vi "Run.vi"(8 "error in (no error)":errorcluster, 9 "s on last turn":dbl, 10 "Maze (0: Empty, -1: Enemy. >0: Teammate":i32[][](array[numeric]), 11 "Expand in":refnum<class "Hungry Wolf.lvclass">) -> (0 "error out":errorcluster, 1 "Direction":T1, 2 "Action":T2, 3 "Expand out":refnum<class "Hungry Wolf.lvclass">, 4 "Replicated":refnum<class "Square.lvclass">)   [LabVIEW 2015, in "Hungry Wolf.lvclass"]
uses:
  Hungry Wolf.lvclass
  Type Defs/Action Enum.ctl
  Type Defs/Direction Enum.ctl
  Square/Square.lvclass
  Hungry Wolf.lvclass/Hungry Wolf.ctl
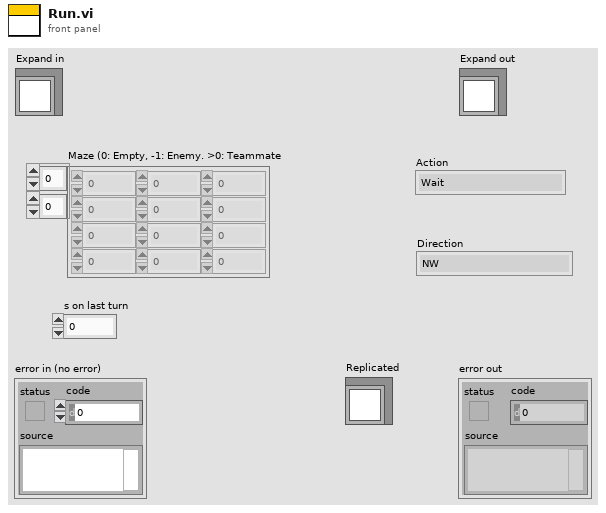
[diagram p1: front panel]
types:
  T1 = typedef "Square.lvclass/Direction Enum.ctl" = enum16{"NW", "N", "NE", "E", "SE", "S", "SW", "W"}
  T2 = typedef "Square.lvclass/Action Enum.ctl" = enum16{"Wait", "Move", "Attack", "Replicate"}
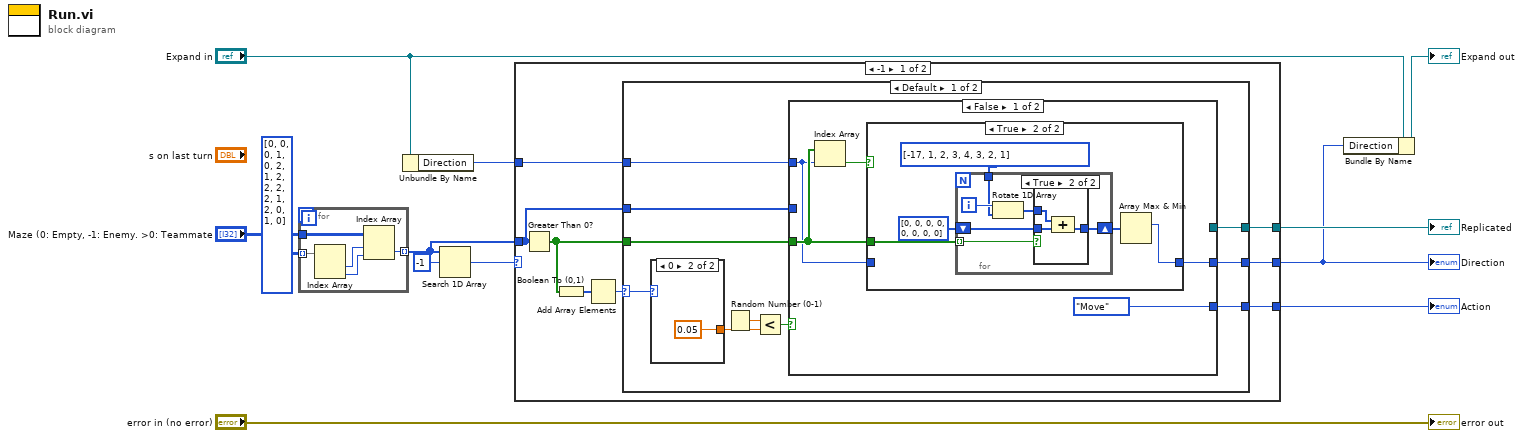
[diagram p0: block diagram]
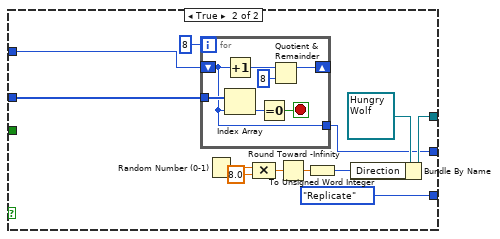
[diagram p5: hidden frame]
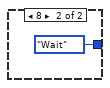
[diagram p6: hidden frame]
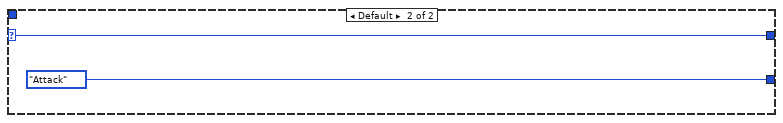
[diagram p7: hidden frame]
diagram:
  n1 = for {
    tunnel: "Maze (0: Empty, -1: Enemy. >0: Teammate" -> [w17]
    tunnel: i32[][] [[0, 0], [0, 1], [0, 2], [1, 2], [2, 2], [2, 1], [2, 0], [1, 0]] -> [w16] mode=indexing
    tunnel: [w13] -> w7 mode=indexing
    n2 = Index Array(array=w16) -> (element #1=w15:i32, element #2=w14:i32)  [unwired: 2 in]
    n3 = Index Array(array=w17, index (row)=w15, index (col)=w14) -> (element=w13:i32)
  }
  n4 = Unbundle By Name("Expand in") -> ("Direction"=w1:T1)
  n5 = Search 1D Array(1D array=w7, element=-1) -> (index of element=w8:i32)  [unwired: 1 in]
  n6 = case shown="-1" w8 {
    selector: w8 -> [_ w78]
    tunnel: [w24 w78] -> w4
    tunnel: [w25 Action_Enum."Attack" ("Action")] -> w5
    tunnel: w7 -> [w21 _]
    tunnel: [w23 _] -> w6
    tunnel: w1 -> [w22 _]
    frame -1 {
      n7 = Greater Than 0?(x=w21) -> (x > 0?=w19:bool[])
      n8 = Boolean To (0,1)(Boolean=w19) -> (0, 1=w20:i16[])
      n9 = Add Array Elements(numeric array=w20) -> (sum=w18:i16)
      n10 = case shown="Default" w18 {
        selector: w18 -> [w27 _]
        tunnel: [w35 Action_Enum."Wait" ("y")] -> w25
        tunnel: [w34 _] -> w24
        tunnel: [w33 _] -> w23
        tunnel: w19 -> [w28 _]
        tunnel: w22 -> [w32 _]
        tunnel: w21 -> [w31 _]
        frame Default {
          n11 = case shown="0" w27 {
            tunnel: [_ 0.05] -> w26
            frame Default {
            }
            frame 0 {
            }
          }
          n12 = Random Number (0-1)() -> (number: 0 to 1=w30:dbl)
          n13 = Less?(x=w30, y=w26) -> (x < y?=w29:bool)
          n14 = case shown="False" w29 {
            tunnel: [Action_Enum."Move" ("y") Action_Enum."Replicate" ("y")] -> w35
            tunnel: [w40 w58] -> w34
            tunnel: [_ w67] -> w33
            tunnel: w32 -> [w37 w60]
            tunnel: w31 -> [_ w59]
            tunnel: w28 -> [w39 _]
            frame False {
              n15 = Index Array(array=w39, index=w37) -> (element=w38:bool)
              n16 = case shown="True" w38 {
                tunnel: [w42 w44] -> w40
                tunnel: w39 -> [_ w43]
                tunnel: w37 -> [w42 _]
                frame False {
                }
                frame True {
                  n17 = for {
                    tunnel: w43 -> [w51] mode=indexing
                    tunnel: i32[] [-17, 1, 2, 3, 4, 3, 2, 1] -> [w52]
                    shift-right: [w49] -> w47
                    shift-left: i32[] [0, 0, 0, 0, 0, 0, 0, 0] -> [w48]
                    i -> [w53]
                    n18 = Rotate 1D Array(1:w52, 2:w53) -> (0:w50:i32[])
                    n19 = case shown="True" w51 {
                      tunnel: w50 -> [_ w57]
                      tunnel: [w54 w56] -> w49
                      tunnel: w48 -> [w54 w55]
                      frame False {
                      }
                      frame True {
                        n20 = Compound Arithmetic op=ADD(w57, w55) -> (w56:i32[])
                      }
                    }
                  }
                  n21 = Array Max & Min(array=w47) -> (max index (indices)=w44:i32)  [unwired: 3 out]
                }
              }
            }
            frame True {
              n22 = for {
                N: 8 -> [_]
                tunnel: w59 -> [w76]
                shift-right: [w72] -> _
                shift-left: w60 -> [w71]
                tunnel: [w71] -> w58
                stop <- w70 stop-if-true
                n23 = Increment(x=w71) -> (x+1=w74:i32)
                n24 = Index Array(array=w76, index=w71) -> (element=w75:i32)
                n25 = Equal To 0?(x=w75) -> (x = 0?=w70:bool)
                n26 = Quotient & Remainder(x=w74, y=8) -> (x-y*floor(x/y)=w72:i32)  [unwired: 1 out]
              }
              n27 = Random Number (0-1)() -> (number: 0 to 1=w63:dbl)
              n28 = Compound Arithmetic op=MULTIPLY(w63, 8.0 ("value")) -> (w65:dbl)
              n29 = Round Toward -Infinity(1:w65) -> (0:w66:dbl)
              n30 = To Unsigned Word Integer(number=w66) -> (unsigned 16bit integer=w62:u16)
              n31 = Bundle By Name(cluster=refnum<class "Hungry Wolf.lvclass"> refnum ("Lone Wolf.lvclass"), "Direction"=w62) -> (w67:refnum<class "Hungry Wolf.lvclass">)
            }
          }
        }
        frame 8 {
        }
      }
    }
    frame Default {
    }
  }
  "Action" <- w5
  "Direction" <- w4
  "Replicated" <- w6
  n32 = Bundle By Name(cluster="Expand in", "Direction"=w4) -> (→"Expand out":refnum<class "Hungry Wolf.lvclass">)
  "error out" <- "error in (no error)"
